vi "Get Plain Text Extension.vi"(8 "error in (no error)":errorcluster caption="错误输入（无错误）", 11 "Gif Image 输入":refnum<class "Gif Image.lvclass"> caption="DNL_LabVIEW Object in") -> (0 "error out":errorcluster caption="错误输出", 3 "Gif Image 输出":refnum<class "Gif Image.lvclass"> caption="DNL_LabVIEW Object out")   [LabVIEW 2011, in "Gif Image.lvclass"]
uses:
  Gif Image.lvclass
  Control/Plain Text Extension.ctl
  Control/ID Charactor.ctl
panel:
  out "Plain Text Extension":T1 {"Plain Text Label(1)" format="0x%02x" items=["Image Seperator"=44, "Extension Introducer"=33, "Graphic Control Label"=249, "Comment Label"=254, "PlainText Label"=1, "Gif Trailor"=59, "Application Label"=255]; "ID(1)" format="0x%02x" items=["Image Seperator"=44, "Extension Introducer"=33, "Graphic Control Label"=249, "Comment Label"=254, "PlainText Label"=1, "Gif Trailor"=59, "Application Label"=255]}
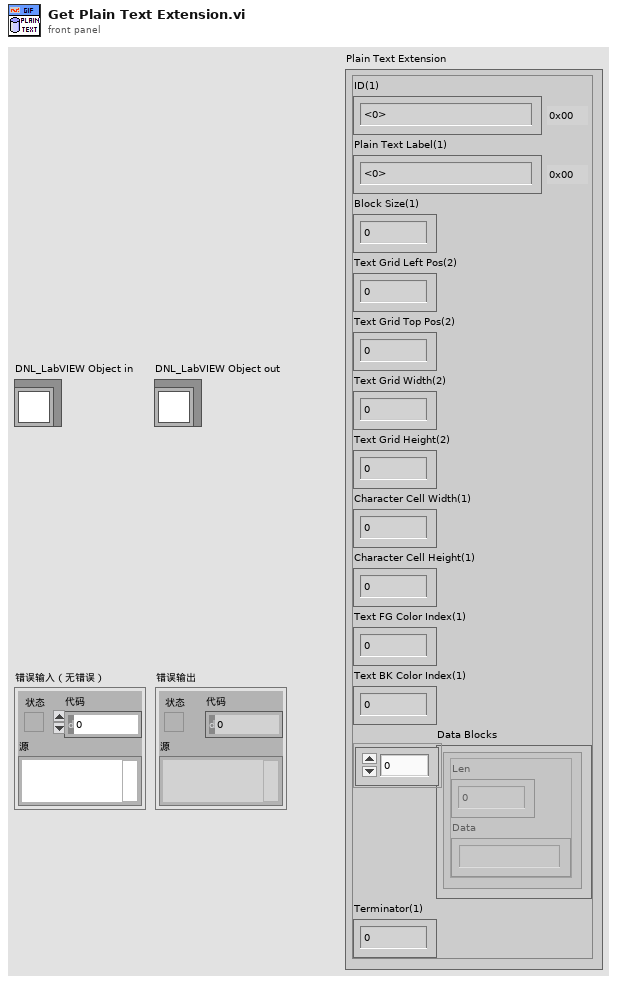
[diagram p1: front panel]
types:
  T1 = typedef "Gif Image.lvclass/Plain Text Extension.ctl" = cluster{"ID(1)":T2, "Plain Text Label(1)":T2, "Block Size(1)":u8, "Text Grid Left Pos(2)":u16, "Text Grid Top Pos(2)":u16, "Text Grid Width(2)":u16, "Text Grid Height(2)":u16, "Character Cell Width(1)":u8, "Character Cell Height(1)":u8, "Text FG Color Index(1)":u8, "Text BK Color Index(1) ":u8, "Data Blocks":cluster{"Len":u8, "Data":string}[], "Terminator(1)":u8}
  T2 = typedef "Gif Image.lvclass/ID Charactor.ctl" = u8
  T3 = enum16{"big-endian, network order", "native, host order", "little-endian"}
  T4 = cluster{"ID(1)":T2, "Plain Text Label(1)":T2, "Block Size(1)":u8, "Text Grid Left Pos(2)":u16, "Text Grid Top Pos(2)":u16, "Text Grid Width(2)":u16, "Text Grid Height(2)":u16, "Character Cell Width(1)":u8, "Character Cell Height(1)":u8, "Text FG Color Index(1)":u8, "Text BK Color Index(1)":u8}
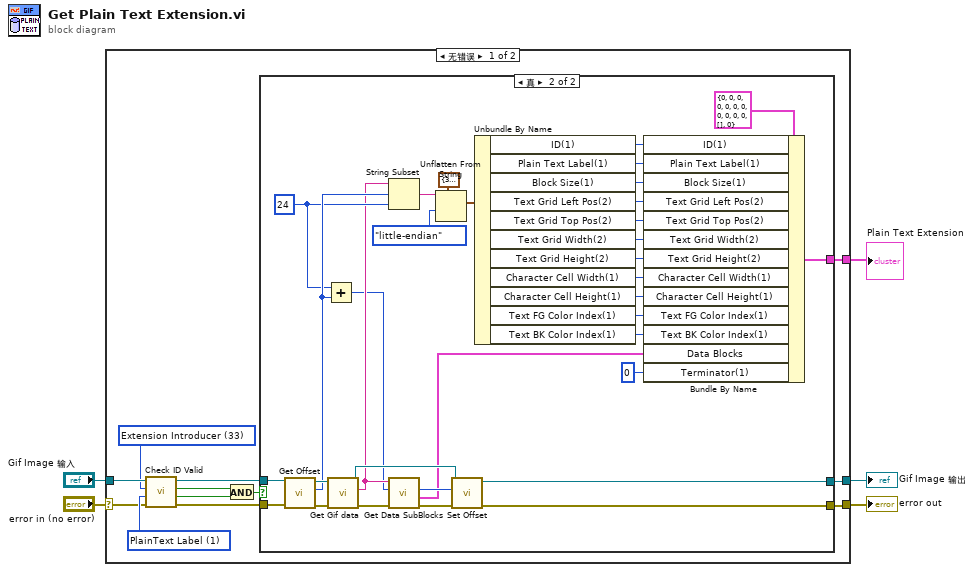
[diagram p0: block diagram]
diagram:
  n1 = case shown="无错误" "error in (no error)" {
    selector: "error in (no error)" -> [w10 w54]
    tunnel: [w8 w54] -> w4
    tunnel: "Gif Image 输入" -> [w17 w53]
    tunnel: [w7 w53] -> w2
    tunnel: [w6 _] -> w1
    frame No Error {
      w15 = T2 1 items=["Image Seperator"=44, "Extension Introducer"=33, "Graphic Control Label"=249, "Comment Label"=254, "PlainText Label"=1, "Gif Trailor"=59, "Application Label"=255] ("Label")
      w16 = T2 33 items=["Image Seperator"=44, "Extension Introducer"=33, "Graphic Control Label"=249, "Comment Label"=254, "PlainText Label"=1, "Gif Trailor"=59, "Application Label"=255] ("ID")
      n2 = call "Check ID Valid.vi"("error in (no error)"=w10, "Label"=w15, "ID"=w16, "Gif Image 输入"=w17) -> ("error out"=w9:errorcluster, "Label Valid"=w13:bool, "ID Valid"=w14:bool, "Gif Image 输出"=w11:refnum<class "Gif Image.lvclass">)  [unwired: 4 in]
      n3 = And(x=w14, y=w13) -> (x .and. y?=w12:bool)
      n4 = case shown="真" w12 {
        tunnel: w11 -> [w18 w52]
        tunnel: w9 -> [w19 w51]
        tunnel: [w19 w45] -> w8
        tunnel: [w18 w44] -> w7
        tunnel: [_ w20] -> w6
        frame False {
        }
        frame True {
          w47 = 24 ("长度（剩余）")
          n5 = call "Get Offset.vi"("error in (no error)"=w51, "Gif Image输入"=w52) -> ("error out"=w50:errorcluster, "Offset"=w48:i32, "Gif Image输出"=w49:refnum<class "Gif Image.lvclass">)  [unwired: 7 in]
          n6 = Add(x=w47, y=w48) -> (x+y=w39:i32)
          n7 = call "Get Gif data.vi"("error in (no error)"=w50, "Gif Image输入"=w49) -> ("error out"=w43:errorcluster, "Gif data"=w41:string, "Gif Image输出"=w46:refnum<class "Gif Image.lvclass">)  [unwired: 7 in]
          n8 = String Subset(string=w41, offset (0)=w48, length (rest)=w47) -> (substring=w38:string)
          n9 = call "Get Data SubBlocks.vi"("错误输入"=w43, "Offset In"=w39, "Gif data in"=w41) -> ("错误输出"=w42:errorcluster, "Data Blocks"=w22:cluster{"Len":u8, "Gif data Out":string}[], "Offset Out"=w40:i32)  [unwired: 5 in, 1 out]
          n10 = Unflatten From String(type=T4 {"ID(1)"=33, "Plain Text Label(1)"=1, "Block Size(1)"=0, "Text Grid Left Pos(2)"=0, "Text Grid Top Pos(2)"=0, "Text Grid Width(2)"=0, "Text Grid Height(2)"=0, "Character Cell Width(1)"=0, "Character Cell Height(1)"=0, "Text FG Color Index(1)"=0, "Text BK Color Index(1)"=0}, binary string=w38, byte order (0:big-endian, network order)=T3."little-endian" ("字节顺序(0:big-endian, network order)")) -> (value=w36:T4)  [unwired: 2 in, 2 out]
          n11 = call "Set Offset.vi"("error in (no error)"=w42, "Offset"=w40, "Gif Image输入"=w46) -> ("error out"=w45:errorcluster, "Gif Image输出"=w44:refnum<class "Gif Image.lvclass">)  [unwired: 7 in]
          n12 = Unbundle By Name(w36) -> ("ID(1)"=w35:T2, "Plain Text Label(1)"=w34:T2, "Block Size(1)"=w33:u8, "Text Grid Left Pos(2)"=w32:u16, "Text Grid Top Pos(2)"=w30:u16, "Text Grid Width(2)"=w29:u16, "Text Grid Height(2)"=w28:u16, "Character Cell Width(1)"=w27:u8, "Character Cell Height(1)"=w26:u8, "Text FG Color Index(1)"=w25:u8, "Text BK Color Index(1)"=w24:u8)
          n13 = Bundle By Name(cluster=T1 {"ID(1)"=0, "Plain Text Label(1)"=0, "Block Size(1)"=0, "Text Grid Left Pos(2)"=0, "Text Grid Top Pos(2)"=0, "Text Grid Width(2)"=0, "Text Grid Height(2)"=0, "Character Cell Width(1)"=0, "Character Cell Height(1)"=0, "Text FG Color Index(1)"=0, "Text BK Color Index(1) "=0, "Data Blocks"=[], "Terminator(1)"=0} ("Plain Text Extension"), "ID(1)"=w35, "Plain Text Label(1)"=w34, "Block Size(1)"=w33, "Text Grid Left Pos(2)"=w32, "Text Grid Top Pos(2)"=w30, "Text Grid Width(2)"=w29, "Text Grid Height(2)"=w28, "Character Cell Width(1)"=w27, "Character Cell Height(1)"=w26, "Text FG Color Index(1)"=w25, "Text BK Color Index(1)"=w24, "Data Blocks"=w22, "Terminator(1)"=u8 0) -> (w20:T1)
        }
      }
    }
    frame Error {
    }
  }
  "error out" <- w4
  "Gif Image 输出" <- w2
  "Plain Text Extension" <- w1
